vi "8164B.Create Message Session.vi"(8 "error in":errorcluster, 10 "stop event":refnum<user-event>) -> (0 "error out":errorcluster, 2 "8164B Message queue":refnum<queue>, 3 "8164B Message Session out":T1)   [LabVIEW 2018]
uses:
  typedefs/8164B.Message Type.ctl
  typedefs/8164.Message Session.ctl
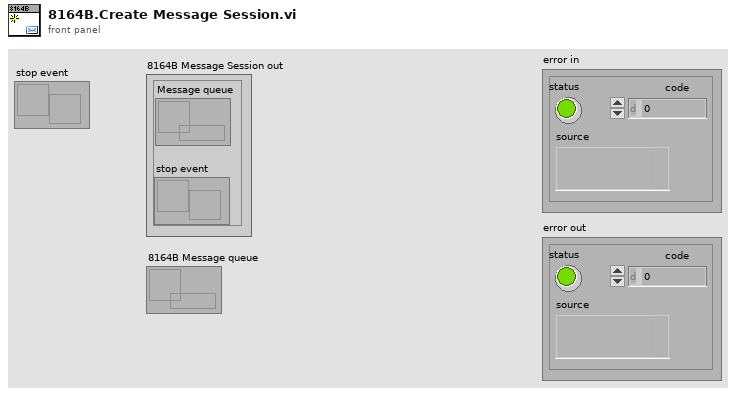
[diagram p1: front panel]
types:
  T1 = typedef "8164.Message Session.ctl" = cluster{"Message queue":refnum<queue>, "stop event":refnum<user-event>}
  T2 = typedef "8164B.Message Type.ctl" = enum16{"meas", "set level", "set gate"}
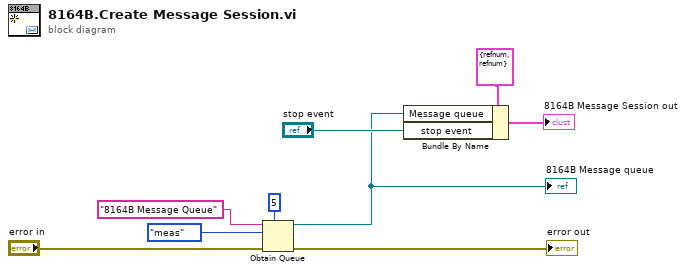
[diagram p0: block diagram]
diagram:
  n1 = Obtain Queue(max queue size (-1, unlimited)=5, name (unnamed)="8164B Message Queue", element data type=8164B.Message_Type."meas" ("8164B.Message type"), error in (no error)="error in") -> (queue out=w2:refnum<queue>, error out=→"error out":errorcluster)  [unwired: 1 in, 1 out]
  "8164B Message queue" <- w2
  n2 = Bundle By Name(cluster=T1 {"Message queue"=refnum, "stop event"=refnum} ("8164B.Message Session"), "Message queue"=w2, "stop event"="stop event") -> (→"8164B Message Session out":T1)
